vi "CRC32-MPEG.vi"(4 "Data In":string) -> (7 "CRC":u32 format="%08x")   [LabVIEW 2020, in "Vecto.lvlib"]
uses:
  Vecto.lvlib
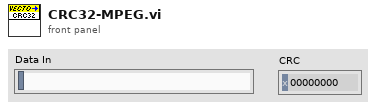
[diagram p1: front panel]
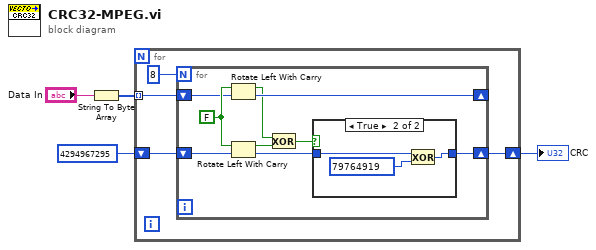
[diagram p0: block diagram]
diagram:
  n1 = String To Byte Array(string="Data In") -> (unsigned byte array=w1:u8[])
  n2 = for {
    shift-right: [w5] -> w2
    shift-left: u32 4294967295 ("Initial CRC") -> [w7]
    tunnel: w1 -> [w6] mode=indexing
    n3 = for {
      N: 8 -> [_]
      shift-right: [w12] -> w5
      shift-left: w7 -> [w10]
      shift-right: [w15] -> _
      shift-left: w6 -> [w16]
      w17 = FALSE ("carry")
      n4 = Rotate Left With Carry(2:w16, 3:w17) -> (0:w15:u8, 1:w14:bool)
      n5 = Rotate Left With Carry(2:w10, 3:w17) -> (0:w9:u32, 1:w11:bool)
      n6 = Exclusive Or(1:w11, 2:w14) -> (0:w13:bool)
      n7 = case shown="True" w13 {
        tunnel: w9 -> [w18 w21]
        tunnel: [w18 w20] -> w12
        frame False {
        }
        frame True {
          n8 = Exclusive Or(1:u32 79764919, 2:w21) -> (0:w20:u32)
        }
      }
    }
  }
  "CRC" <- w2
